vi "Load Test Image File.vi"(8 "error in (no error)":errorcluster, 11 "name or relative path":string="HDMI_Image_Test.png") -> (0 "error out":errorcluster, 2 "Test Image":picture, 3 "Test Image Data":u32[][](array[numeric]) format="%x")   [LabVIEW 2011]
uses:
  <vilib>/picture/picture.llb/imagedata.ctl
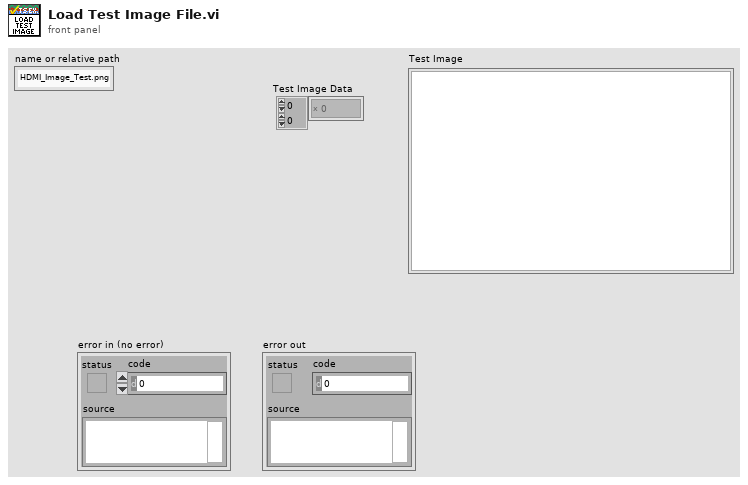
[diagram p1: front panel]
types:
  T1 = typedef "imagedata.ctl" = cluster{"image type":i32, "image depth":i32, "image":u8[], "mask":u8[], "colors":u32[], "Rectangle":cluster{"left":i16, "top":i16, "right":i16, "bottom":i16}}
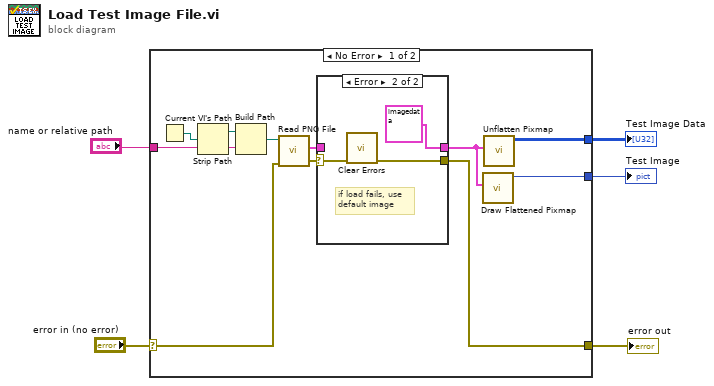
[diagram p0: block diagram]
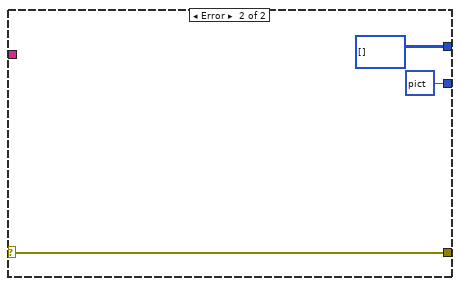
[diagram p3: hidden frame]
diagram:
  n1 = case shown="No Error" "error in (no error)" {
    selector: "error in (no error)" -> [w6 w24]
    tunnel: "name or relative path" -> [w13 _]
    tunnel: [w12 u32[][] [] ("24-bit pixmap")] -> w4
    tunnel: [w11 picture data[5B] ("new picture")] -> w3
    tunnel: [w7 w24] -> w2
    frame No Error {
      n2 = Current VI's Path() -> (path=w16:path)
      n3 = Strip Path(path=w16) -> (stripped path=w15:path)  [unwired: 1 out]
      n4 = Build Path(base path=w15, name or relative path=w13) -> (appended path=w14:path)
      n5 = call <vilib>:"Read PNG File.vi"("error in (no error)"=w6, "path to PNG file"=w14) -> ("error out"=w9:errorcluster, "image data"=w10:T1)  [unwired: 7 in, 1 out]
      n6 = case shown="Error" w9 {
        selector: w9 -> [w17 w20]
        tunnel: w10 -> [w18 _]
        tunnel: [w18 T1 {"image type"=0, "image depth"=24, "image"=array[191040 elements], "mask"=[], "colors"=[], "Rectangle"={"left"=0, "top"=0, "right"=320, "bottom"=199}} ("image data")] -> w8
        tunnel: [w17 w19] -> w7
        frame No Error {
        }
        frame Error {
          # "if load fails, use\ndefault image"
          n7 = call <vilib>:"Clear Errors.vi"("error in (no error)"=w20) -> ("error out"=w19:errorcluster)  [unwired: 6 in]
        }
      }
      n8 = call <vilib>:"Draw Flattened Pixmap.vi"("image data"=w8) -> ("new picture"=w11:picture)  [unwired: 8 in]
      n9 = call <vilib>:"Unflatten Pixmap.vi"("image data"=w8) -> ("24-bit pixmap"=w12:u32[][])  [unwired: 4 in, 6 out]
    }
    frame Error {
    }
  }
  "error out" <- w2
  "Test Image Data" <- w4
  "Test Image" <- w3
